vi "DEBUG.vi"(4 "Debug Tag (none)":string, 5 "Dev DEBUG? (f)":bool) -> (1 "DEBUG?":bool)   [LabVIEW 2011]
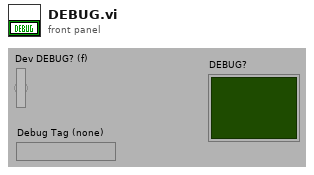
[diagram p1: front panel]
types:
  T1 = enum32{"invalid app kind", "Development System", "Run Time System", "Student Edition", "Embedded LabVIEW", "Evaluation", "Custom"}
  T2 = typedef "NI_LVConfig.lvlib/Config Data RefNum.ctl" = refnum<k1>
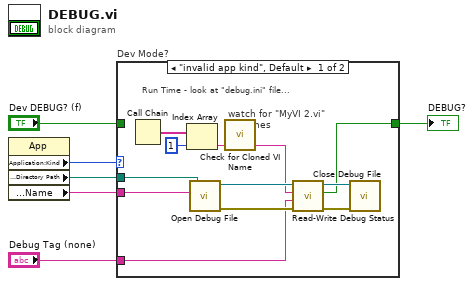
[diagram p0: block diagram]
diagram:
  n1 = property class="App"() -> ("Application:Kind"=w6:T1, "Application:Directory Path"=w2:path, "Application:Name"=w1:string)  [unwired: 2 in, 2 out]
  n2 = case "Dev Mode?" shown="\"invalid app kind\", Default" w6 {
    tunnel: "Dev DEBUG? (f)" -> [_ w19]
    tunnel: [w12 w19] -> w4
    tunnel: "Debug Tag (none)" -> [w9 _]
    tunnel: w2 -> [w18 _]
    tunnel: w1 -> [w17 _]
    frame "invalid app kind", Default {
      # "watch for \"MyVI 2.vi\"\nVI clones"
      # "Run Time - look at \"debug.ini\" file..."
      n3 = Call Chain() -> (call chain=w16:string[])
      n4 = Index Array(array=w16, index=1) -> (element=w8:string)
      n5 = call "Open Debug File.vi"("App Name (\"\")"=w17, "App Folder (Empty)"=w18) -> ("error out"=w10:errorcluster, "Debug Ref"=w14:T2)  [unwired: 1 in, 3 out]
      n6 = call "Check for Cloned VI Name.vi"("Possible Clone VI Name"=w8) -> ("Root VI Name"=w7:string)  [unwired: 4 out]
      n7 = call "Read-Write Debug Status.vi"("error in (no error)"=w10, "Debug Tag (\"\")"=w9, "Debugged VI Name (\"\")"=w7, "Debug Ref"=w14) -> ("error out"=w11:errorcluster, "DEBUG?"=w12:bool, "dup Debug Ref"=w13:T2)  [unwired: 1 out]
      n8 = call "Close Debug File.vi"("error in (no error)"=w11, "Debug refnum"=w13) -> ()  [unwired: 6 out]
    }
    frame "Development System" {
      # "Just read input boolean..."
    }
  }
  "DEBUG?" <- w4
